vi "LeftClick.vi"(6 "Double Click":bool, 7 "Table History ref":refnum<vi>, 8 "error in (no error)":errorcluster, 9 "Table CtlRef In":refnum<vi>, 10 "Cell Position":T1, 11 "DigitalCol in":refnum<class "DigitalCol.lvclass">) -> (0 "error out":errorcluster, 1 "Table CtlRef Out":refnum<vi>, 2 "Discard?":bool, 3 "DigitalCol out":refnum<class "DigitalCol.lvclass">, 5 "Button":u16=1)   [LabVIEW 2013, in "DigitalCol.lvclass"]
doc: "Left-clicking a 0/1 will toggle value and update the color appropriately. Double-click brings up edit so user can add a variable. Single click of a character other than 0 or 1 will also bring up edit.\nThis VI is read-only w.r.t. column data."
uses:
  DigitalCol.lvclass
  <vilib>/Utility/miscctls.llb/LVRowAndColumnTypeDef.ctl
  TypeDefs/TableHistory.ctl
  TypeDefs/TableArray.ctl
  Column/Column.lvclass/Column.ctl
  Column/Column.lvclass
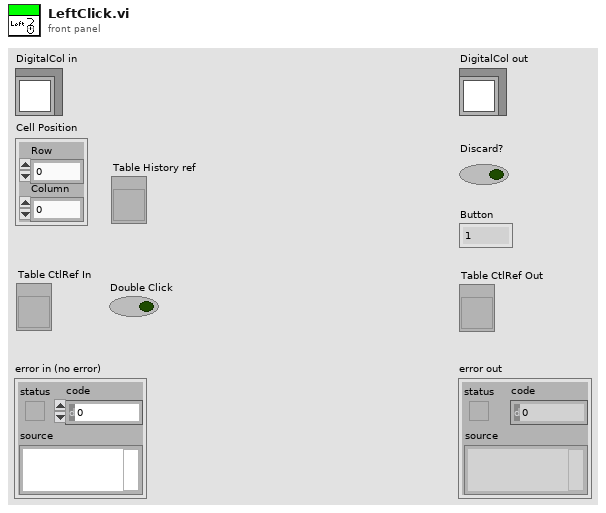
[diagram p1: front panel]
types:
  T1 = typedef "LVRowAndColumnTypeDef.ctl" = cluster{"Row":i32, "Column":i32}
  T2 = typedef "TableHistory.ctl" = cluster{"OldTable Array":T3, "Undo pointer":i32}
  T3 = typedef "TableArray.ctl" = cluster{"OldTable":string[][]}[]
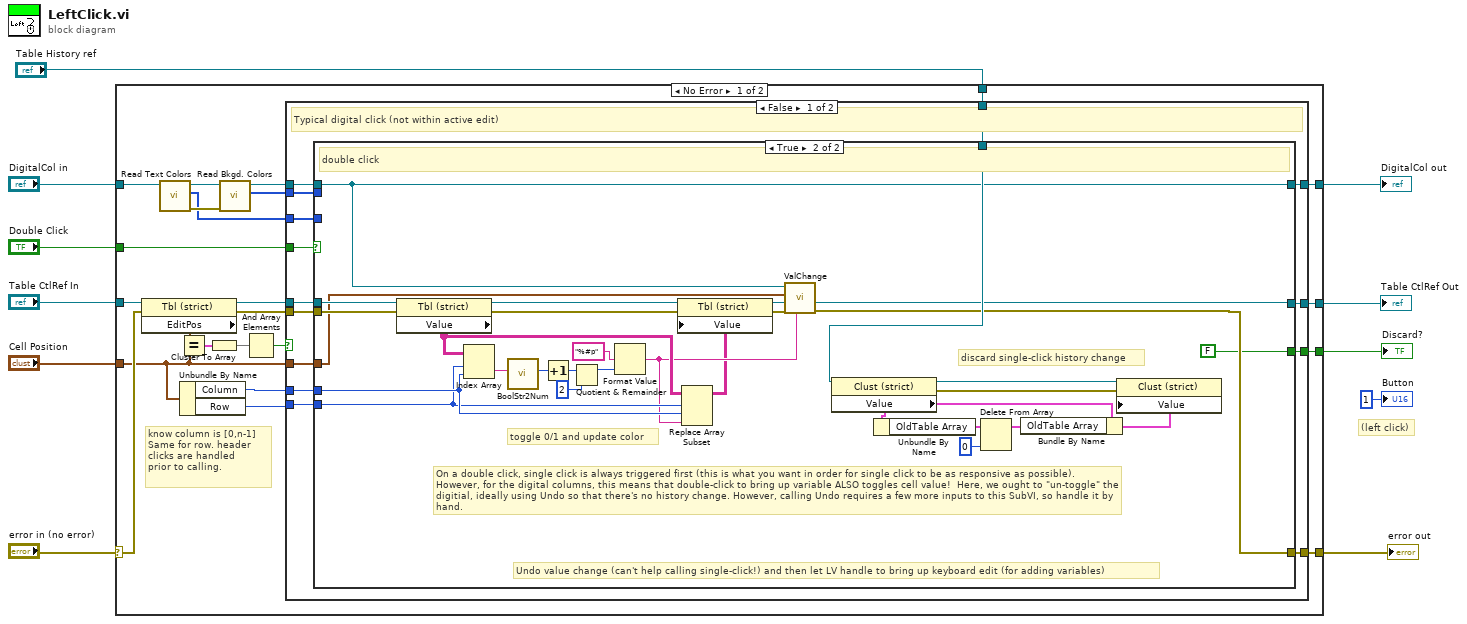
[diagram p0: block diagram]
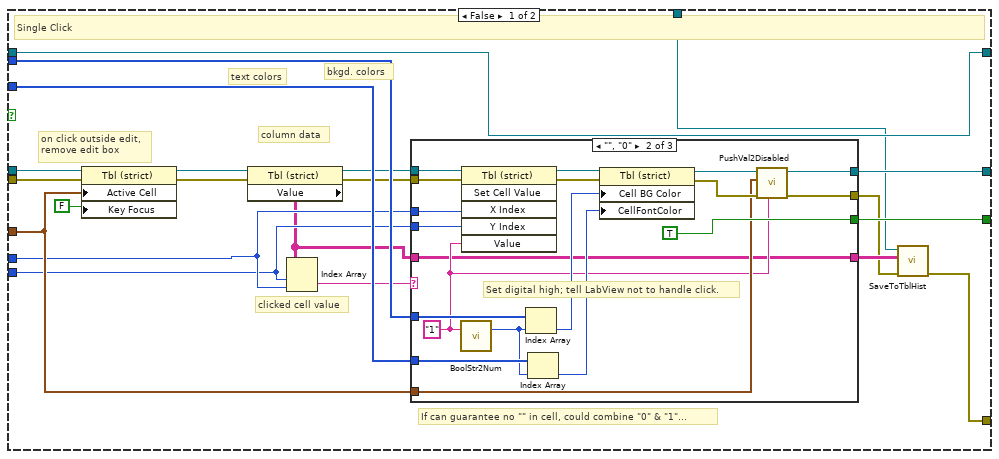
[diagram p2: hidden frame]
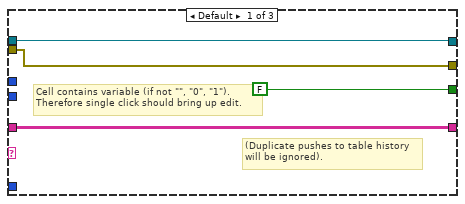
[diagram p3: hidden frame]
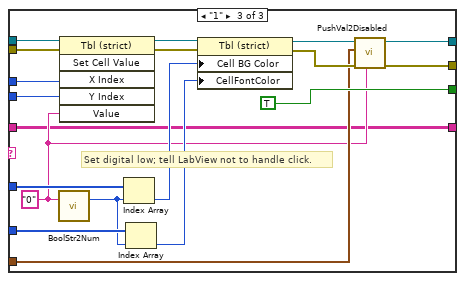
[diagram p4: hidden frame]
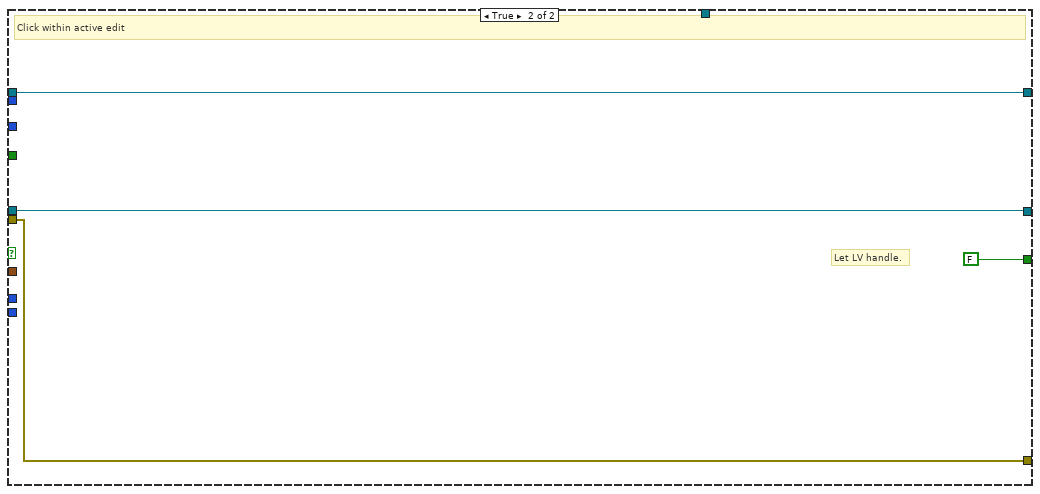
[diagram p5: hidden frame]
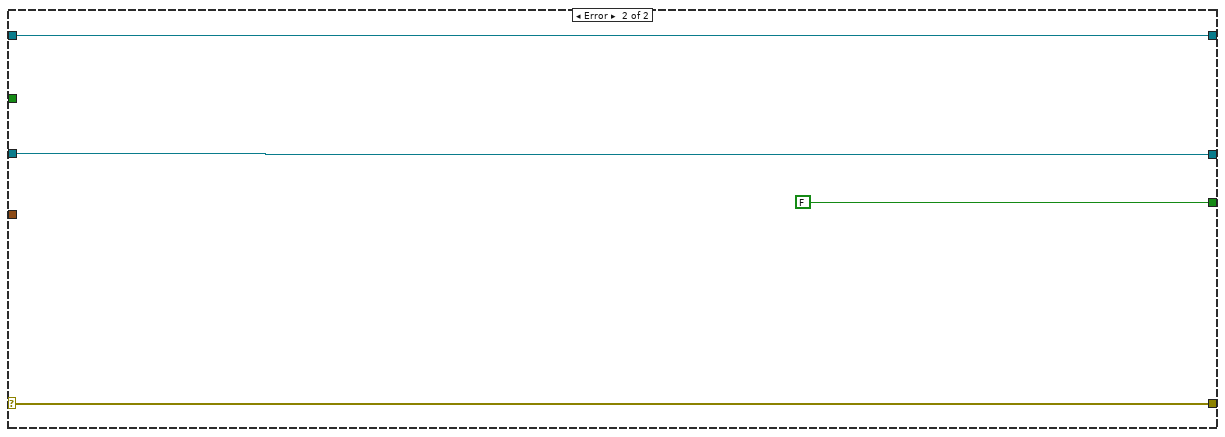
[diagram p6: hidden frame]
diagram:
  # "(left click)"
  n1 = case shown="No Error" "error in (no error)" {
    selector: "error in (no error)" -> [w26 w148]
    tunnel: [w33 w148] -> w6
    tunnel: [w30 w147] -> w10
    tunnel: "DigitalCol in" -> [w18 w147]
    tunnel: "Cell Position" -> [w12 _]
    tunnel: [w34 FALSE] -> w7
    tunnel: "Table CtlRef In" -> [w28 w145]
    tunnel: [w32 w145] -> w8
    tunnel: "Double Click" -> [w31 _]
    tunnel: "Table History ref" -> [w29 _]
    frame No Error {
      # "know column is [0,n-1]\nSame for row. header\nclicks are handled\nprior to calling."
      n2 = property class="Tbl (strict)"(reference=w28, error in=w26) -> (reference out=w27:refnum<vi>, error out=w25:errorcluster, "EditPos"=w24:T1)
      n3 = call "Read Text Colors.vi"("Column in"=w18) -> ("error out"=w20:errorcluster, "Text Colors"=w15:u32[], "Column out"=w19:refnum<class "DigitalCol.lvclass">)  [unwired: 8 in]
      n4 = Equal?(x=w24, y=w12) -> (x = y?=w23:cluster{"Row":bool, "Column":bool})
      n5 = Unbundle By Name(w12) -> ("Column"=w14:i32, "Row"=w13:i32)
      n6 = Cluster To Array(cluster=w23) -> (array=w22:bool[])
      n7 = call "Read Bkgd. Colors.vi"("error in (no error)"=w20, "Column in"=w19) -> ("Bkgd. Colors"=w16:u32[], "Column out"=w17:refnum<class "DigitalCol.lvclass">)  [unwired: 7 in, 1 out]
      n8 = And Array Elements(Boolean array=w22) -> (logical AND=w21:bool)
      n9 = case shown="False" w21 {
        tunnel: [w48 FALSE] -> w34
        tunnel: [w47 w143] -> w33
        tunnel: [w46 w144] -> w32
        tunnel: w31 -> [w45 _]
        tunnel: w17 -> [w44 w142]
        tunnel: [w43 w142] -> w30
        tunnel: w29 -> [w42 _]
        tunnel: w27 -> [w41 w144]
        tunnel: w25 -> [w40 w143]
        tunnel: w12 -> [w39 _]
        tunnel: w16 -> [w38 _]
        tunnel: w15 -> [w37 _]
        tunnel: w14 -> [w36 _]
        tunnel: w13 -> [w35 _]
        frame False {
          # "Typical digital click (not within active edit)"
          n10 = case shown="True" w45 {
            tunnel: w39 -> [w61 w131]
            tunnel: w40 -> [w64 w137]
            tunnel: [w69 FALSE] -> w48
            tunnel: [w65 w136] -> w47
            tunnel: w41 -> [w62 w139]
            tunnel: [w68 w138] -> w46
            tunnel: w44 -> [w67 w132]
            tunnel: [w67 w132] -> w43
            tunnel: w42 -> [w66 w140]
            tunnel: w38 -> [w59 _]
            tunnel: w37 -> [w58 _]
            tunnel: w36 -> [w56 w134]
            tunnel: w35 -> [w55 w133]
            frame False {
              # "If can guarantee no \"\" in cell, could combine \"0\" & \"1\"..."
              # "column data"
              # "clicked cell value"
              # "on click outside edit,\nremove edit box"
              # "text colors"
              # "bkgd. colors"
              # "Single Click"
              n11 = property on="Property Node" class="Tbl (strict)"(reference=w62, error in=w64, "Active Cell"=w61, "Key Focus"=FALSE) -> (reference out=w63:refnum<vi>, error out=w57:errorcluster)
              n12 = property on="Property Node" class="Tbl (strict)"(reference=w63, error in=w57) -> (reference out=w54:refnum<vi>, error out=w52:errorcluster, "Value"=w51:string[][])
              n13 = Index Array(array=w51, index (row)=w55, index (col)=w56) -> (element=w53:string)
              n14 = case shown="\"\", \"0\"" w53 {
                tunnel: w56 -> [_ w88 w107]
                tunnel: w55 -> [_ w87 w106]
                tunnel: [w71 w80 w99] -> w49
                tunnel: [FALSE TRUE TRUE] -> w69
                tunnel: w54 -> [w72 w90 w109]
                tunnel: [w72 w78 w97] -> w68
                tunnel: w52 -> [w71 w86 w105]
                tunnel: w59 -> [_ w85 w104]
                tunnel: w58 -> [_ w84 w103]
                tunnel: w61 -> [_ w77 w96]
                tunnel: w51 -> [w70 w74 w93]
                tunnel: [w70 w74 w93] -> w50
                frame Default {
                  # "(Duplicate pushes to table history\nwill be ignored)."
                  # "Cell contains variable (if not \"\", \"0\", \"1\").\nTherefore single click should bring up edit."
                }
                frame "", "0" {
                  w75 = "1" ("Value")
                  # "Set digital high; tell LabView not to handle click."
                  n15 = call "BoolStr2Num.vi"("Boolean string"=w75) -> ("number"=w76:i32)  [unwired: 10 in]
                  n16 = invoke on="Invoke Node" class="Tbl (strict)" method="Set Cell Value"(reference=w90, error in=w86, "X Index"=w88, "Y Index"=w87, "Value"=w75) -> (reference out=w89:refnum<vi>, error out=w92:errorcluster)  [unwired: 1 in, 4 out]
                  n17 = Index Array(array=w85, index=w76) -> (element=w83:u32)
                  n18 = Index Array(array=w84, index=w76) -> (element=w82:u32)
                  n19 = property on="Property Node" class="Tbl (strict)"(reference=w89, error in=w92, "Cell BG Color"=w83, "CellFontColor"=w82) -> (reference out=w79:refnum<vi>, error out=w81:errorcluster)
                  n20 = call "PushVal2Disabled.vi"("Value"=w75, "error in (no error)"=w81, "Cell Position"=w77, "Table CtlRef In"=w79) -> ("error out"=w80:errorcluster, "Table CtlRef Out"=w78:refnum<vi>)  [unwired: 5 in, 1 out]
                }
                frame "1" {
                  w94 = "0" ("Value")
                  # "Set digital low; tell LabView not to handle click."
                  n21 = call "BoolStr2Num.vi"("Boolean string"=w94) -> ("number"=w95:i32)  [unwired: 10 in]
                  n22 = invoke on="Invoke Node" class="Tbl (strict)" method="Set Cell Value"(reference=w109, error in=w105, "X Index"=w107, "Y Index"=w106, "Value"=w94) -> (reference out=w108:refnum<vi>, error out=w111:errorcluster)  [unwired: 1 in, 4 out]
                  n23 = Index Array(array=w104, index=w95) -> (element=w102:u32)
                  n24 = Index Array(array=w103, index=w95) -> (element=w101:u32)
                  n25 = property on="Property Node" class="Tbl (strict)"(reference=w108, error in=w111, "Cell BG Color"=w102, "CellFontColor"=w101) -> (reference out=w98:refnum<vi>, error out=w100:errorcluster)
                  n26 = call "PushVal2Disabled.vi"("Value"=w94, "error in (no error)"=w100, "Cell Position"=w96, "Table CtlRef In"=w98) -> ("error out"=w99:errorcluster, "Table CtlRef Out"=w97:refnum<vi>)  [unwired: 5 in, 1 out]
                }
              }
              n27 = call "SaveToTblHist.vi"("error in (no error)"=w49, "OldTable (reset)"=w50, "Table History ref"=w66) -> ("error out"=w65:errorcluster)  [unwired: 8 in]
            }
            frame True {
              # "toggle 0/1 and update color"
              # "discard single-click history change"
              # "On a double click, single click is always triggered first (this is what you want in order for single click to be as responsive as possible). However, for the digital columns, this means that double-click to bring up variable ALSO toggles cell value!  Here, we ought to \"un-toggle\" the digitial, ideally using Undo so that there's no history change. However, calling Undo requires a few more inputs to this SubVI, so handle it by hand."
              # "Undo value change (can't help calling single-click!) and then let LV handle to bring up keyboard edit (for adding variables)"
              # "double click"
              n28 = property class="Tbl (strict)"(reference=w139, error in=w137) -> (reference out=w116:refnum<vi>, error out=w114:errorcluster, "Value"=w118:string[][])
              n29 = Index Array(array=w118, index (row)=w133, index (col)=w134) -> (element=w123:string)
              n30 = call "BoolStr2Num.vi"("Boolean string"=w123) -> ("number"=w122:i32)  [unwired: 10 in]
              n31 = Increment(x=w122) -> (x+1=w121:i32)
              n32 = Quotient & Remainder(x=w121, y=2) -> (x-y*floor(x/y)=w119:i32)  [unwired: 1 out]
              n33 = Format Value(format string="%#p", value (0)=w119) -> (output string=w117:string)  [unwired: 1 in]
              n34 = Replace Array Subset(array=w118, new element=w117, index (row)=w133, index (col)=w134) -> (w113:string[][])
              n35 = property class="Tbl (strict)"(reference=w116, error in=w114, "Value"=w113) -> (reference out=w138:refnum<vi>, error out=w115:errorcluster)
              n36 = call-dynamic "ValChange.vi"("Value"=w117, "error in (no error)"=w115, "Table CtlRef In"=w138, "Cell Position"=w131, "DigitalCol in"=w132) -> ("error out"=w136:errorcluster)  [unwired: 4 in, 2 out]
              n37 = property class="Clust (strict)"(reference=w140) -> (reference out=w130:refnum<vi>, error out=w129:errorcluster, "Value"=w126:T2)  [unwired: 1 in]
              n38 = Unbundle By Name(w126) -> ("OldTable Array"=w128:T3)
              n39 = Delete From Array(array=w128, index=0) -> (array with subset deleted=w125:T3)  [unwired: 1 in, 1 out]
              n40 = Bundle By Name(cluster=w126, "OldTable Array"=w125) -> (w124:T2)
              n41 = property class="Clust (strict)"(reference=w130, error in=w129, "Value"=w124) -> ()  [unwired: 2 out]
            }
          }
        }
        frame True {
          # "Let LV handle."
          # "Click within active edit"
        }
      }
    }
    frame Error {
    }
  }
  "error out" <- w6
  "DigitalCol out" <- w10
  "Discard?" <- w7
  "Table CtlRef Out" <- w8
  "Button" <- u16 1 ("Button")
